vi "grab_qrcode_numpy.vi"() -> ()   [LabVIEW 2018]
uses:
  0460686a-1f5f-4a7d-b7f5-93a42d0cd41c.vi
panel:
  out "filename":string
  in  "stop":bool
  out "Input QR Code":picture
  out "Output QR Code":picture
  out "return value":cluster{"found":i32, "decode data":string}
  in  "Output image filename":string="decode.png"
  in  "QR Code Image Path":string="qrcode_src"
  # "Free QR code generator website"
  # "https://www.the-qrcode-generator.com/"
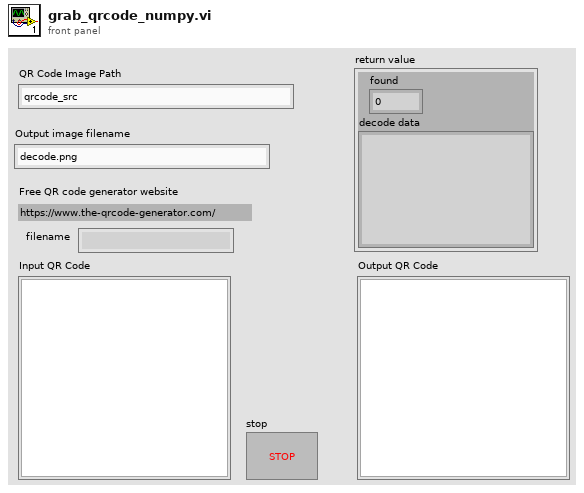
[diagram p1: front panel]
types:
  T1 = typedef "imagedata.ctl" = cluster{"image type":i32, "image depth":i32, "image":u8[], "mask":u8[], "colors":u32[], "Rectangle":cluster{"left":i16, "top":i16, "right":i16, "bottom":i16}}
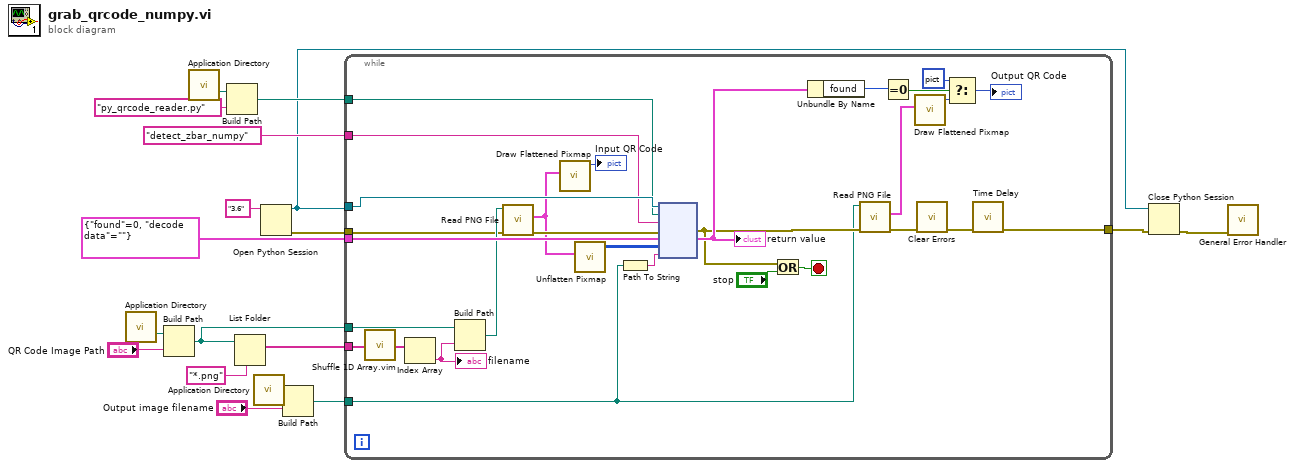
[diagram p0: block diagram]
diagram:
  n1 = call <vilib>:"Application Directory.vi"() -> ("Application Directory"=w10:path)
  n2 = Build Path(base path=w10, name or relative path="QR Code Image Path") -> (appended path=w8:path)
  n3 = call <vilib>:"Application Directory.vi"() -> ("Application Directory"=w16:path)
  n4 = Build Path(base path=w16, name or relative path="py_qrcode_reader.py" ("module filename")) -> (appended path=w14:path)
  n5 = List Folder(path=w8, pattern="*.png") -> (filenames=w13:string[])  [unwired: 2 in, 3 out]
  n6 = call <vilib>:"Application Directory.vi"() -> ("Application Directory"=w3:path)
  n7 = Open Python Session(python version="3.6" ("Python version")) -> (session out=w6:refnum<k35>, error out=w7:errorcluster)  [unwired: 2 in]
  n8 = Build Path(base path=w3, name or relative path="Output image filename") -> (appended path=w1:path)
  n9 = while {
    tunnel: w6 -> [w47]
    tunnel: w7 -> [w24]
    tunnel: "detect_zbar_numpy" ("function name") -> [w46]
    tunnel: cluster{"found":i32, "decode data":string} {"found"=0, "decode data"=""} -> [w45]
    tunnel: w14 -> [w43]
    tunnel: w8 -> [w36]
    tunnel: w13 -> [w41]
    tunnel: [w32] -> w12
    tunnel: w1 -> [w19]
    stop <- w38 stop-if-true
    n10 = call "Shuffle 1D Array.vim"("array"=w41) -> ("shuffled array"=w40:string[])  [unwired: 4 in]
    n11 = Index Array(array=w40) -> (element=w35:string)  [unwired: 1 in]
    "filename" <- w35
    n12 = Build Path(base path=w36, name or relative path=w35) -> (appended path=w25:path)
    n13 = call <vilib>:"Read PNG File.vi"("error in (no error)"=w24, "path to PNG file"=w25) -> ("error out"=w23:errorcluster, "image data"=w20:T1)  [unwired: 7 in, 1 out]
    n14 = call <vilib>:"Draw Flattened Pixmap.vi"("image data"=w20) -> ("new picture"=→"Input QR Code":picture)  [unwired: 8 in]
    n15 = call <vilib>:"Unflatten Pixmap.vi"("image data"=w20) -> ("24-bit pixmap"=w22:u32[][])  [unwired: 4 in, 6 out]
    n16 = Path To String(path=w19) -> (string=w33:string)
    n17 = node(w47, w43, w46, w23, w45, w22, w33) -> (w21:errorcluster, w31:cluster{"found":i32, "decode data":string})  [unwired: 2 in, 3 out]
    "return value" <- w31
    n18 = Or(x=w21, y="stop") -> (x .or. y?=w38:bool)
    n19 = Unbundle By Name(w31) -> ("found"=w30:i32)
    n20 = call <vilib>:"Read PNG File.vi"("error in (no error)"=w21, "path to PNG file"=w19) -> ("error out"=w37:errorcluster, "image data"=w44:T1)  [unwired: 7 in, 1 out]
    n21 = Equal To 0?(x=w30) -> (x = 0?=w29:bool)
    n22 = call <vilib>:"Draw Flattened Pixmap.vi"("image data"=w44) -> ("new picture"=w27:picture)  [unwired: 8 in]
    n23 = call <vilib>:"Clear Errors.vi"("error in (no error)"=w37) -> ("error out"=w34:errorcluster)  [unwired: 5 in, 1 out]
    n24 = Select(t=picture data[5B] ("picture"), s=w29, f=w27) -> (s? t:f=→"Output QR Code":picture)
    n25 = call "Time Delay"("error in (no error)"=w34) -> ("error out"=w32:errorcluster)  [unwired: 10 in]
  }
  n26 = Close Python Session(session in=w6, error in=w12) -> (11:w11:errorcluster)
  n27 = call <vilib>:"General Error Handler.vi"("error in (no error)"=w11) -> ()  [unwired: 10 in, 5 out]
